vi "feedback_linearization.vi"() -> ()   [LabVIEW 2019]
uses:
  <vilib>/myRIO/Common/Instrument Driver Framework/myRIO v1.0/IRQ/typedefs/DI IRQ Type.ctl
  <vilib>/userDefined/High Color/nirio_resource_hc.ctl
  <vilib>/Platform/TimedLoop/XDataNode/timing_clust.ctl
  <vilib>/Platform/TimedLoop/XDataNode/nitl_modes.ctl
  <vilib>/Platform/TimedLoop/XDataNode/wakeup.ctl
  <vilib>/myRIO/Common/Instrument Driver Framework/myRIO v1.0/PWM/vis/myRIO v1.0 Close PWM.vi
  <vilib>/myRIO/Common/Instrument Driver Framework/myRIO v1.0/PWM/vis/myRIO v1.0 Unreserve PWM.vi
  <vilib>/myRIO/Common/Instrument Driver Framework/myRIO v1.0/PWM/vis/myRIO v1.0 Build MUX Configuration PWM.vi
  <vilib>/myRIO/Common/Instrument Driver Framework/myRIO v1.0/Resource Manager/vis/myRIO v1.0 Unreserve Channel List.vi
  <vilib>/myRIO/Common/Instrument Driver Framework/myRIO v1.0/Resource Manager/vis/myRIO v1.0 Create Configuration List.vi
  <vilib>/myRIO/Common/Instrument Driver Framework/myRIO v1.0/Resource Manager/vis/myRIO v1.0 Unreserve Channel.vi
  <vilib>/myRIO/Common/Instrument Driver Framework/myRIO v1.0/Resource Manager/vis/myRIO v1.0 Build Mutex Name.vi
  <vilib>/Utility/file.llb/Read Delimited Spreadsheet (DBL).vi
  rpm.vi
  ISR.vi
  <vilib>/myRIO/Common/Instrument Driver Framework/myRIO v1.0/IRQ/vis/myRIO v1.1 Register DI IRQ.vi
  <vilib>/Utility/file.llb/Write Delimited Spreadsheet (DBL).vi
  <vilib>/Utility/error.llb/Error Cluster From Error Code.vi
  <vilib>/myRIO/Common/Instrument Driver Framework/myRIO v1.0/PWM/vis/myRIO v1.0 Write PWM.vi
  <vilib>/myRIO/Common/Instrument Driver Framework/myRIO v1.0/PWM/vis/myRIO v1.0 Shutdown PWM.vi
  <vilib>/myRIO/Common/Instrument Driver Framework/myRIO v1.0/Resource Manager/vis/myRIO v1.0 Configure IO.vi
  <vilib>/myRIO/Common/Instrument Driver Framework/Utilities/vis/Configuration Manager.vi
  <vilib>/myRIO/Common/Instrument Driver Framework/Utilities/vis/IO Manager.vi
  <vilib>/myRIO/Common/Instrument Driver Framework/myRIO v1.0/myRIO v1.0 Close.vi
  <vilib>/myRIO/Common/Instrument Driver Framework/myRIO v1.0/IRQ/vis/myRIO v1.0 Reserve IRQ.vi
  <vilib>/myRIO/Common/Instrument Driver Framework/Utilities/vis/FPGA Ref Manager.vi
  <vilib>/myRIO/Express VI/IRQ/IRQ Express VI.xnode
  <vilib>/myRIO/Instrument Drivers/IRQ/IO IRQ/vis/myRIO Register DI IRQ.xnode
  <vilib>/myRIO/Common/Instrument Driver Framework/myRIO v1.0/IRQ/typedefs/Callback VI Ref.ctl
  <vilib>/platform/TimedLoop/XDataNode/XDataNode.xnode
  <vilib>/Platform/TimedLoop/XDataNode/XDNodeRunTimeDep.lvlib
  <vilib>/myRIO/Instrument Drivers/Onboard IO/PWM/PWM.lvlib
  <vilib>/Utility/Variable/NI_VariableUtilities.lvlib
  <vilib>/myRIO/Instrument Drivers/IRQ/IO IRQ/IO IRQ.lvlib
panel:
  out "N":i32
  out "i":i32
  out "Max. Iteration Duration":i64
  out "error out (no error) 2":errorcluster
  out "Iteration Duration":i64
  out "omega_vec":dbl[](array[numeric])
  out "Interrupt On":bool
  in  "RPM Inst Data":path=path "/tmp/log.csv"
  out "Omega":dbl[](graph)
  in  "error in (no error)":errorcluster
  out "Np":dbl
  out "ft":dbl
  in  "Input Data":path=path "/tmp/log.csv"
  in  "del_u":dbl=0.15
  in  "u_nominal":dbl=0.55
  out "Finished late":bool
  out "Acquisition State":bool
  in  "Run Time (s)":dbl
  in  "Sampling \nFrequency (Hz)":dbl
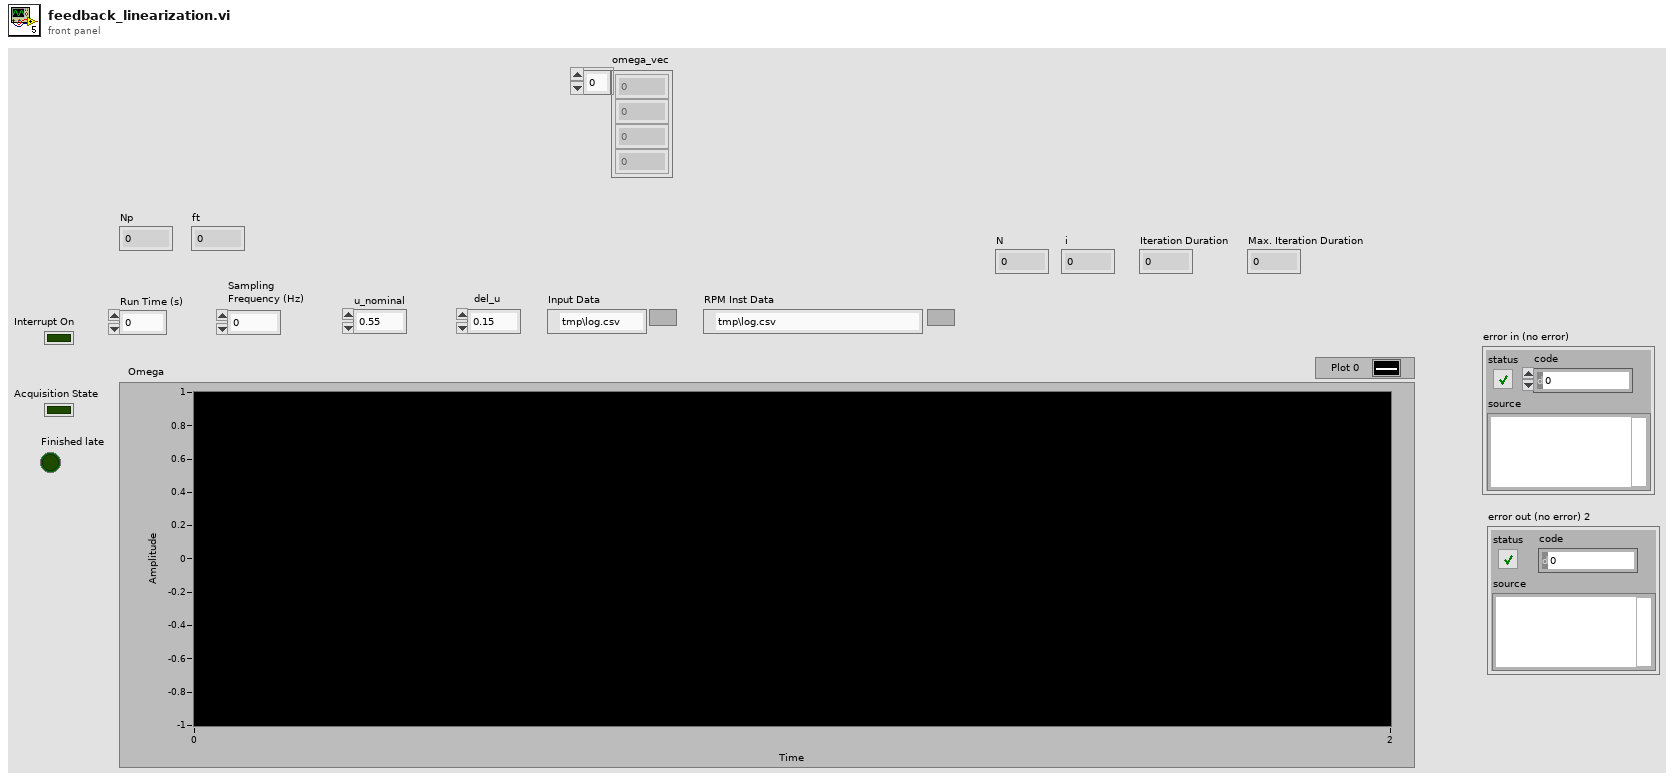
[diagram p1: front panel]
types:
  T1 = typedef "PWM.lvlib/PWM Reference.ctl" = cluster{"myRIO Reference":T2, "PWM Channels Enum":T6, "PWM Configuration":T7}
  T2 = typedef "myRIO Generic Hardware Reference.ctl" = cluster{"myRIO Model":T3, "myRIO Hardware Reference":T4}
  T3 = typedef "Hardware Version Enum.ctl" = enum16{"Unknown", "myRIO-1900", "myRIO-1950", "roboRIO", "NI ELVIS RIO CM", "ELVIS III"}
  T4 = typedef "myRIO v1.0 Reference.ctl" = cluster{"Generic FPGA Reference":T5, "Allow multiple opens":bool}
  T5 = typedef "Generic FPGA Reference.ctl" = refnum<k20>
  T6 = typedef "PWM Channels Enum.ctl" = enum16{"Not Connected", "C/PWM0", "C/PWM1", "A/PWM0", "A/PWM1", "A/PWM2", "A/PWM3", "A/PWM4", "A/PWM5", "A/PWM6", "A/PWM7", "A/PWM8", "A/PWM9", "A/PWM10", "A/PWM11", "A/PWM12", "A/PWM13", "A/PWM14", "A/PWM15", "A/PWM16", "A/PWM17", "A/PWM18", "A/PWM19", "B/PWM0", "B/PWM1", "B/PWM2", "B/PWM3", "B/PWM4", "B/PWM5", "B/PWM6", "B/PWM7", "B/PWM8", "B/PWM9", "B/PWM10", "B/PWM11", "B/PWM12", "B/PWM13", "B/PWM14", "B/PWM15", "B/PWM16", "B/PWM17", "B/PWM18", "B/PWM19", "PWM/PWM0", "PWM/PWM1", "PWM/PWM2", "PWM/PWM3", "PWM/PWM4", "PWM/PWM5", "PWM/PWM6", "PWM/PWM7", "PWM/PWM8", "PWM/PWM9"}
  T7 = typedef "PWM.lvlib/PWM Configuration.ctl" = cluster{"Frequency":dbl, "Duty Cycle":dbl}
  T8 = typedef "XDNodeRunTimeDep.lvlib/timing_clust.ctl" = cluster{"Expected End [f-1]":u64, "Actual End [f-1]":u64, "Finished Late? [f-1]":bool, "Expected End [i-1]":u64, "Actual End [i-1]":u64, "Finished Late? [i-1]":bool, "Expected Start [i]":u64, "Actual Start [i]":u64, "Expected Start [f]":u64, "Actual Start [f]":u64, "Source Name":string, "Structure Name":string, "Period":i64, "Deadline":i64, "Offset":i64, "Start":i64, "Priority":i32, "Timeout":i32, "Mode":T9, "Wakeup Reason":T10, "Error":errorcluster, "Source Type":string, "Secondary Source Type":string, "Global End Time":u64, "Global Start Time":u64, "Frame Duration":u64, "Iteration Duration":u64, "Assigned CPU":i32, "I/O Scan Engine Mode":u32}
  T9 = typedef "XDNodeRunTimeDep.lvlib/nitl_modes.ctl" = enum32{"No Change", "Process missed periods, maintain original phase", "Discard missed periods, maintain original phase", "Process missed periods, ignore original phase", "Discard missed periods, ignore original phase"}
  T10 = typedef "XDNodeRunTimeDep.lvlib/wakeup.ctl" = enum32{"Normal", "Aborted", "Asynchronous wakeup", "Timing source error", "Timed loop error", "Timeout"}
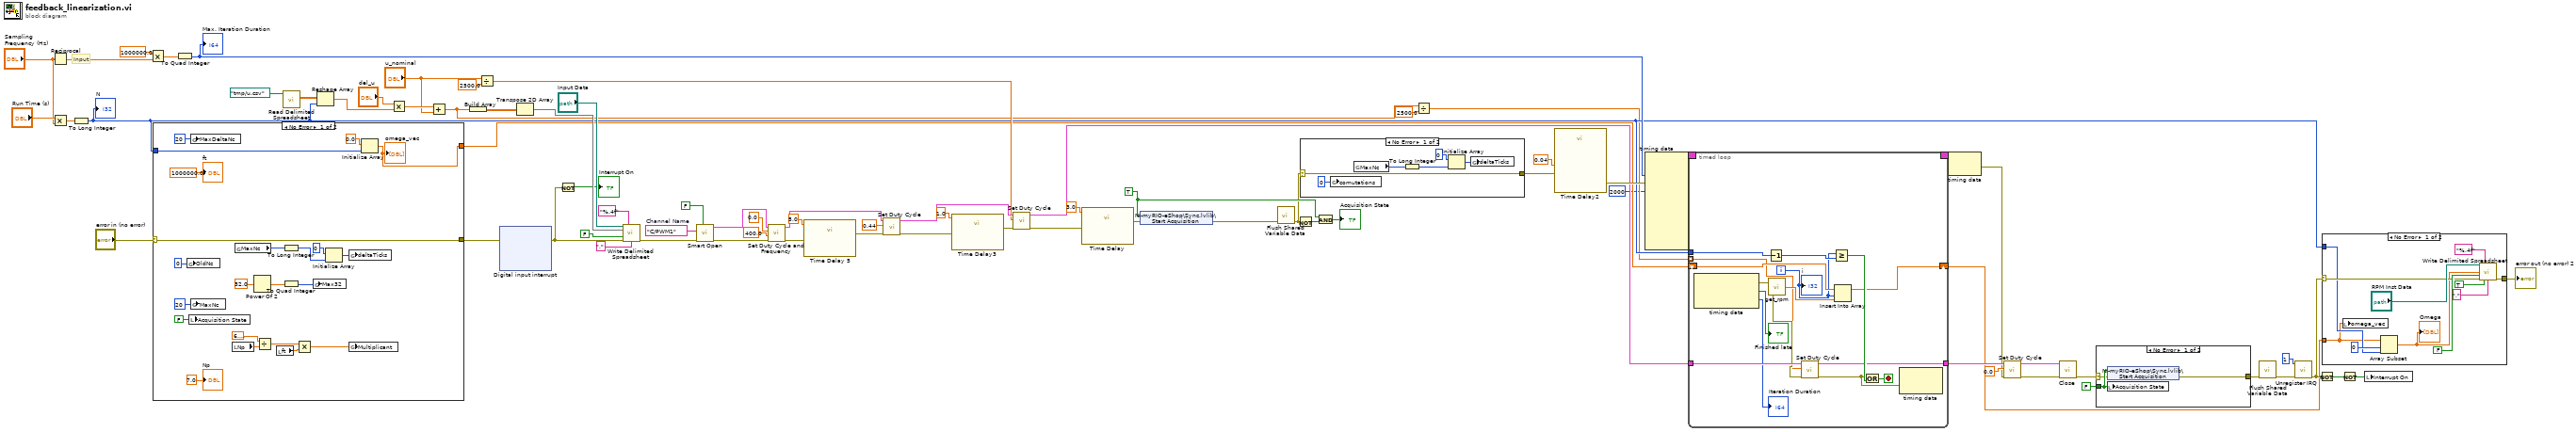
[diagram p0: block diagram]
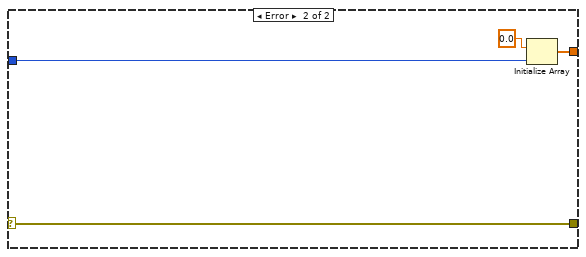
[diagram p5: hidden frame]
diagram:
  w66 = tag "C/PWM1"  # Channel Name
  w45 = TRUE ("Acquisition State")
  # "Input"
  n1 = Reciprocal(x="Sampling \nFrequency (Hz)") -> (1/x=w28:dbl)
  n2 = Multiply(x="Run Time (s)", y="Sampling \nFrequency (Hz)") -> (x*y=w68:dbl)
  n3 = To Long Integer(number=w68) -> (32bit integer=w11:i32)
  "N" <- w11
  n4 = Multiply(x=1000000.0, y=w28) -> (x*y=w36:dbl)
  n5 = case shown="No Error" "error in (no error)" {
    selector: "error in (no error)" -> [w95 w102]
    tunnel: [w95 w102] -> w42
    tunnel: w11 -> [w82 w99]
    tunnel: [w77 w100] -> w9
    frame No Error {
      n6 = global write "rpm.vi" "OldNc"(i64 0 ("MaxNc")) -> ()
      n7 = local write "Acquisition State"(FALSE ("Acquisition State")) -> ()
      n8 = global write "rpm.vi" "MaxDeltaNc"(i64 20 ("MaxDeltaNc")) -> ()
      n9 = global write "rpm.vi" "MaxNc"(i64 20 ("MaxNc")) -> ()
      n10 = local read "Np"() -> (w91:dbl)
      n11 = global read "rpm.vi" "MaxNc"() -> (w79:i64)
      n12 = Power Of 2(x=32.0) -> (2^x=w97:dbl)
      n13 = Divide(x=6.283185307179586, y=w91) -> (x/y=w90:dbl)
      n14 = local read "ft"() -> (w89:dbl)
      n15 = To Long Integer(number=w79) -> (32bit integer=w78:i32)
      n16 = To Quad Integer(1:w97) -> (0:w88:i64)
      n17 = Multiply(x=w90, y=w89) -> (x*y=w98:dbl)
      n18 = global write "rpm.vi" "Max32"(w88) -> ()
      n19 = Initialize Array(i64 0, w78) -> (w80:i64[])
      n20 = global write "rpm.vi" "deltaTicks"(w80) -> ()
      n21 = global write "rpm.vi" "Multiplicant"(w98) -> ()
      n22 = Initialize Array(0.0 ("element"), w82) -> (w77:dbl[])
      "omega_vec" <- w77
      "Np" <- 7.0 ("Numeric")
      "ft" <- 1000000.0 ("ft")
    }
    frame Error {
      n23 = Initialize Array(0.0 ("element"), w99) -> (w100:dbl[])
    }
  }
  n24 = To Quad Integer(1:w36) -> (0:w35:i64)
  "Max. Iteration Duration" <- w35
  n25 = call-poly <vilib>:"Read Delimited Spreadsheet.vi"("file path (dialog if empty)"=path "/tmp/u.csv") -> ("all rows"=w55:dbl[][])  [unwired: 9 in, 5 out]
  n26 = Reshape Array(w55, w11) -> (w54:dbl[])
  n27 = Multiply(x="del_u", y=w54) -> (x*y=w69:dbl[])
  n28 = Add(x=w69, y="u_nominal") -> (x+y=w3:dbl[])
  n29 = Build Array(w3) -> (w70:dbl[][])
  n30 = Divide(x="u_nominal", y=2500.0) -> (x/y=w15:dbl)
  n31 = xnode "Digital input interrupt"("error in (no error)"=w42) -> ("error out"=w33:errorcluster)
  n32 = Transpose 2D Array(2D array=w70) -> (transposed array=w71:dbl[][])
  n33 = Not(x=w33) -> (.not. x?=→"Interrupt On":bool)
  n34 = call-poly <vilib>:"Write Delimited Spreadsheet.vi"("file path (dialog if empty)"="Input Data", "format (%.3f)"="%.4f", "2D data"=w71, "append to file? (new file:F)"=FALSE, "error in (no error)"=w33, "delimiter (\\t)"="," ("delimiter (\\t)")) -> ("error out"=w62:errorcluster)  [unwired: 8 in, 1 out]
  n35 = call <vilib>:"Smart Open.vi"("Allow multiple opens?"=FALSE, "error in (no error)"=w62, "Channel Name"=w66) -> ("error out"=w64:errorcluster, "PWM Ref Out"=w65:T1)  [unwired: 7 in]
  n36 = call <vilib>:"Set Duty Cycle and Frequency.vi"("error in (no error)"=w64, "Frequency [Hz]"=400.0, "Duty Cycle"=0.0, "PWM Ref In"=w65) -> ("error out"=w31:errorcluster, "PWM Ref Out"=w20:T1)  [unwired: 5 in]
  n37 = call "Time Delay 5"("error in (no error)"=w31, "Delay Time (s)"=5.0) -> ("error out"=w21:errorcluster)  [unwired: 9 in]
  n38 = call <vilib>:"Set Duty Cycle.vi"("error in (no error)"=w21, "Duty Cycle"=0.44, "PWM Ref In"=w20) -> ("error out"=w24:errorcluster, "PWM Ref Out"=w18:T1)  [unwired: 6 in]
  n39 = call "Time Delay3"("error in (no error)"=w24, "Delay Time (s)"=1.0) -> ("error out"=w19:errorcluster)  [unwired: 9 in]
  n40 = call <vilib>:"Set Duty Cycle.vi"("error in (no error)"=w19, "Duty Cycle"=w15, "PWM Ref In"=w18) -> ("error out"=w29:errorcluster, "PWM Ref Out"=w30:T1)  [unwired: 6 in]
  n41 = call "Time Delay"("error in (no error)"=w29, "Delay Time (s)"=3.0) -> ("error out"=w57:errorcluster)  [unwired: 9 in]
  n42 = shared-variable "NI-myRIO-eShop\\Sync.lvlib\\Start Acquisition"(w45, error in=w57) -> (error out=w61:errorcluster)
  n43 = call <vilib>:"Flush Shared Variable Data.vi"("error in (no error)"=w61) -> ("error out"=w26:errorcluster)  [unwired: 10 in]
  n44 = Not(x=w26) -> (.not. x?=w25:bool)
  n45 = case shown="No Error" w26 {
    selector: w26 -> [w107 w109]
    tunnel: [w107 w109] -> w39
    frame No Error {
      n46 = global write "rpm.vi" "comutations"(i64 0 ("comutations")) -> ()
      n47 = global read "rpm.vi" "MaxNc"() -> (w104:i64)
      n48 = To Long Integer(number=w104) -> (32bit integer=w103:i32)
      n49 = Initialize Array(i64 0, w103) -> (w105:i64[])
      n50 = global write "rpm.vi" "deltaTicks"(w105) -> ()
    }
    frame Error {
    }
  }
  n51 = And(x=w45, y=w25) -> (x .and. y?=→"Acquisition State":bool)
  n52 = Divide(x=w3, y=2500.0) -> (x/y=w2:dbl[])
  n53 = call "Time Delay2"("error in (no error)"=w39, "Delay Time (s)"=0.04) -> ("error out"=w52:errorcluster)  [unwired: 9 in]
  n54 = node-c288(w35, w52, 2000 ("Priority")) -> (w76:T8)  [unwired: 7 in]
  n55 = timed-loop {
    timing: w76 -> [_]
    timing-out: [_] -> w75
    tunnel: w2 -> [w114] mode=indexing
    tunnel: w30 -> [w125]
    tunnel: w11 -> [w116]
    tunnel: [w122] -> w48
    shift-right: [w117] -> w10
    shift-left: w9 -> [w118]
    i -> [w112]
    stop <- w124 stop-if-true
    n56 = node-c288() -> (w121:errorcluster, →"Finished late":bool, →"Iteration Duration":i64)  [unwired: 1 in]
    n57 = Decrement(x=w116) -> (x-1=w115:i32)
    n58 = call "get_rpm.vi"("error in (no error)"=w121) -> ("RPM"=w119:dbl, "error out"=w120:errorcluster)
    n59 = call <vilib>:"Set Duty Cycle.vi"("error in (no error)"=w120, "Duty Cycle"=w114, "PWM Ref In"=w125) -> ("error out"=w113:errorcluster, "PWM Ref Out"=w122:T1)  [unwired: 6 in]
    n60 = Greater Or Equal?(x=w112, y=w115) -> (x >= y?=w123:bool)
    n61 = Insert Into Array(array=w118, index=w112, new element=w119) -> (w117:dbl[])
    n62 = Or(x=w113, y=w123) -> (x .or. y?=w124:bool)
    n63 = node-c288(w113) -> ()  [unwired: 1 in, 1 out]
    "i" <- w112
  }
  n64 = node-c288(w75) -> (w47:errorcluster)
  n65 = call <vilib>:"Set Duty Cycle.vi"("error in (no error)"=w47, "Duty Cycle"=0.0, "PWM Ref In"=w48) -> ("error out"=w6:errorcluster, "PWM Ref Out"=w7:T1)  [unwired: 6 in]
  n66 = call <vilib>:"Close.vi"("error in (no error)"=w6, "PWM Ref In"=w7) -> ("error out"=w5:errorcluster)  [unwired: 9 in]
  n67 = case shown="No Error" w5 {
    selector: w5 -> [w133 w136]
    tunnel: [w135 w136] -> w60
    tunnel: FALSE ("Start Acquisition") -> [w134 _]
    frame No Error {
      n68 = shared-variable "NI-myRIO-eShop\\Sync.lvlib\\Start Acquisition"(w134, error in=w133) -> (error out=w135:errorcluster)
      n69 = local write "Acquisition State"(w134) -> ()
    }
    frame Error {
    }
  }
  n70 = call <vilib>:"Flush Shared Variable Data.vi"("error in (no error)"=w60) -> ("error out"=w40:errorcluster)  [unwired: 10 in]
  n71 = call <vilib>:"Unregister IRQ.vi"("error in (no error)"=w40, "IRQ Number"=u8 1) -> ("error out"=w13:errorcluster)  [unwired: 9 in]
  n72 = Not(x=w13) -> (.not. x?=w17:bool)
  n73 = case shown="No Error" w13 {
    selector: w13 -> [w142 w148]
    tunnel: [w141 w148] -> w12
    tunnel: w11 -> [w138 _]
    tunnel: w10 -> [w137 _]
    frame No Error {
      n74 = local write "omega_vec"(w137) -> ()
      n75 = Array Subset(array=w137, index=0, length=w138) -> (w140:dbl[])
      "Omega" <- w140
      n76 = call-poly <vilib>:"Write Delimited Spreadsheet.vi"("file path (dialog if empty)"="RPM Inst Data", "format (%.3f)"="%.4f", "1D data"=w140, "append to file? (new file:F)"=FALSE, "error in (no error)"=w142, "transpose? (no:F)"=TRUE, "delimiter (\\t)"="," ("delimiter (\\t)")) -> ("error out"=w141:errorcluster)  [unwired: 7 in, 1 out]
    }
    frame Error {
    }
  }
  "error out (no error) 2" <- w12
  n77 = Not(x=w17) -> (.not. x?=w16:bool)
  n78 = local write "Interrupt On"(w16) -> ()
